vi "background writer.vi"(0 "dictionary":T1, 1 "command queue":refnum<k33>, 2 "response from processor":refnum<k33>, 3 "output type order":T3[](array[typedef]), 5 "logging path":path, 7 "backup directory":path, 9 "cache allocation":T2, 10 "LogRotate":refnum<class "LogRotate.lvclass">=refnum, 11 "scans per write":u16=20, 12 "dictionary group names":T1, 13 "enable channel (bool)":i32, 14 "has enable channel":bool) -> (15 "error out":errorcluster)   [LabVIEW 2015, in "TDMS datalogger runtime.lvclass"]
uses:
  TDMS datalogger runtime.lvclass
  <vilib>/NI/Tag Bus/tag/Data Type.ctl
  data cache.ctl
  <vilib>/NI/Tag Bus/dictionary/full data dictionary.ctl
  message to background process.ctl
  control enum.ctl
  <vilib>/NI/Tag Bus/table/data table.ctl
  response from background process.ctl
  response enum.ctl
  <vilib>/NI/LogRotate/LogRotate.lvclass
  writer state enum.ctl
  <vilib>/NI/Tag Bus/table/data table.lvlib
  <vilib>/NI/Tag Bus/tag/tag descriptor.lvclass
  <vilib>/NI/Tag Bus/dictionary/data dictionary.lvclass
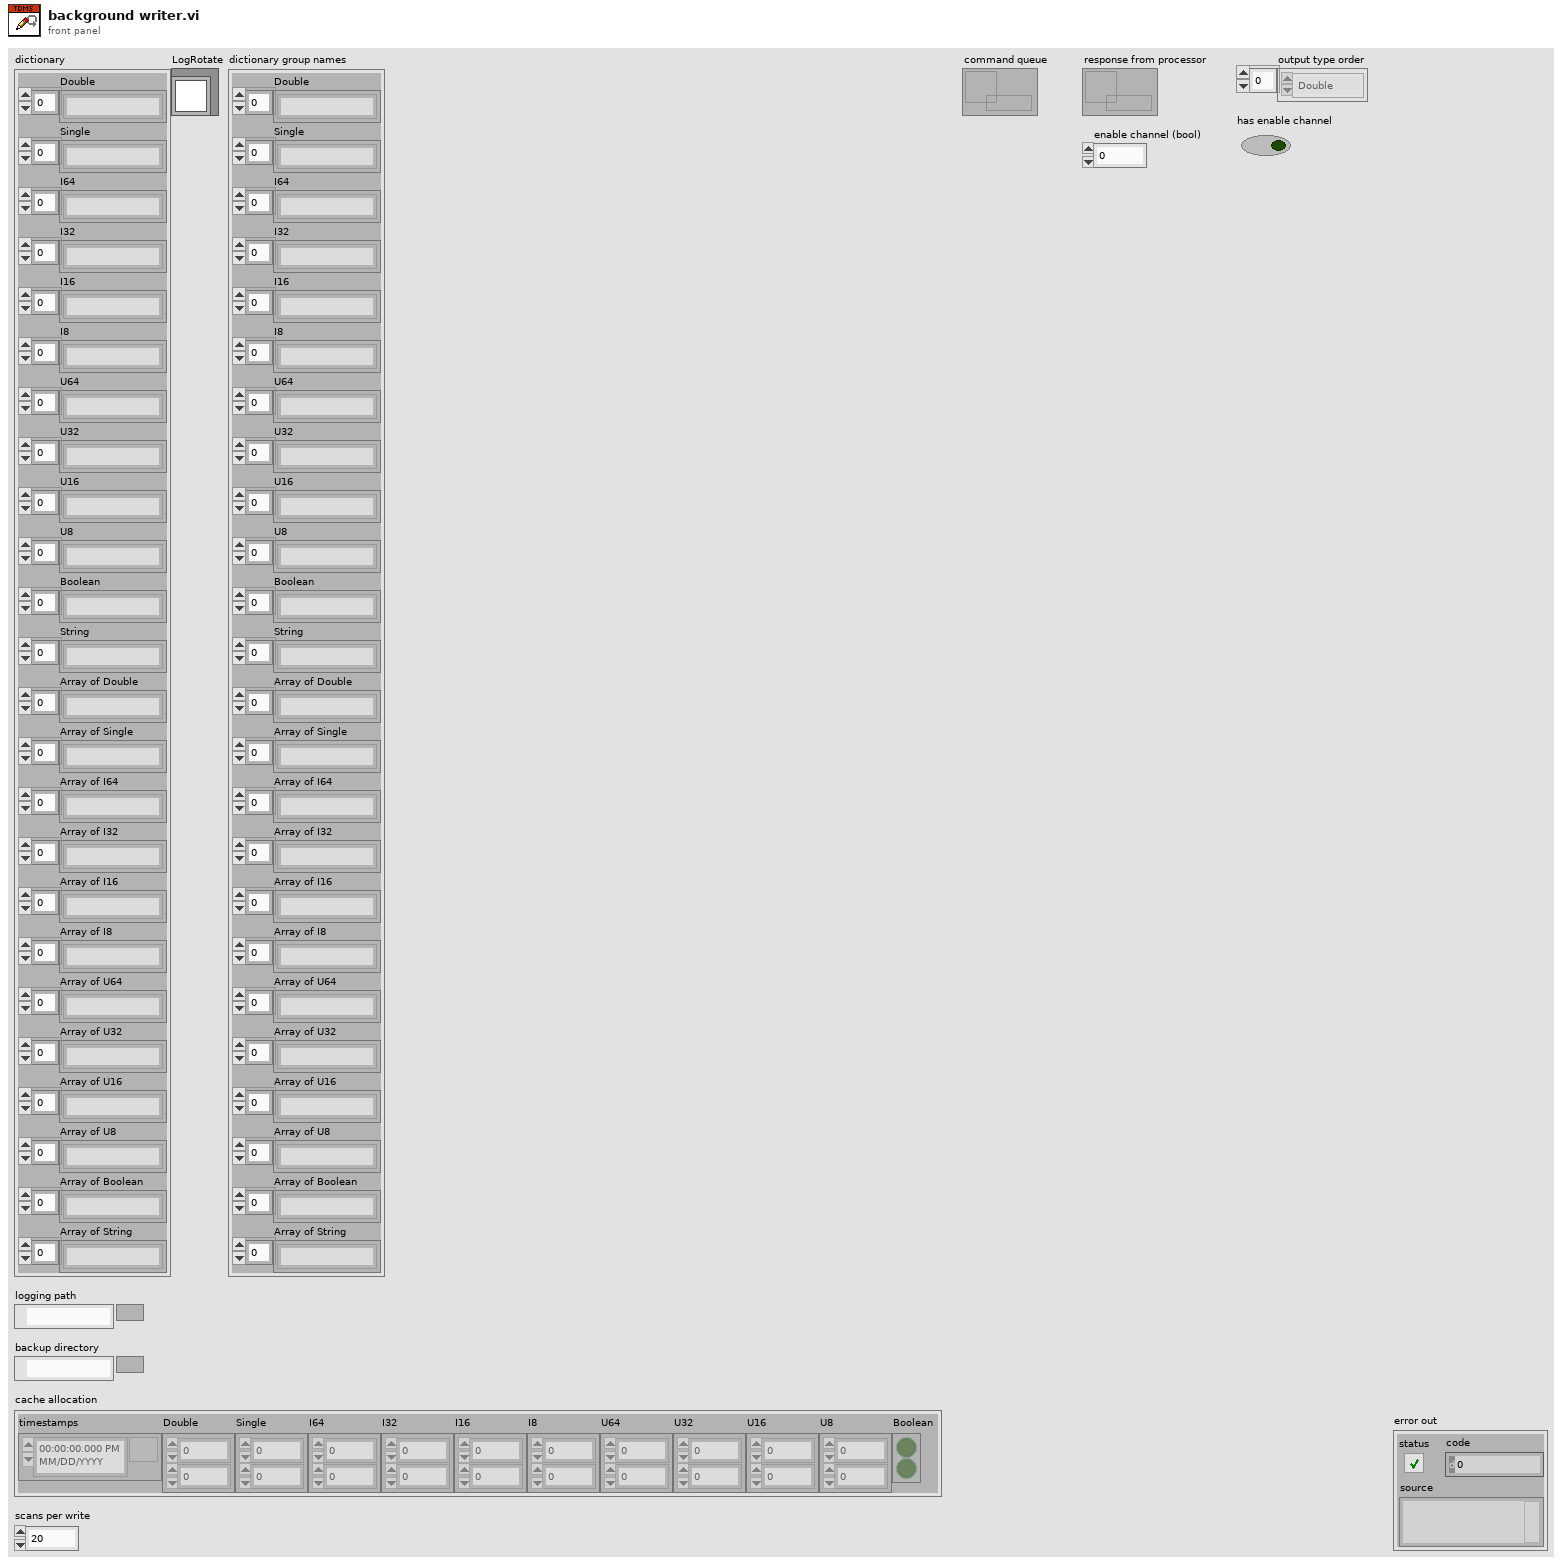
[diagram p1: front panel]
types:
  T1 = typedef "tag bus.lvlib/data dictionary.lvclass/full data dictionary.ctl" = cluster{"Double":string[], "Single":string[], "I64":string[], "I32":string[], "I16":string[], "I8":string[], "U64":string[], "U32":string[], "U16":string[], "U8":string[], "Boolean":string[], "String":string[], "Array of Double":string[], "Array of Single":string[], "Array of I64":string[], "Array of I32":string[], "Array of I16":string[], "Array of I8":string[], "Array of U64":string[], "Array of U32":string[], "Array of U16":string[], "Array of U8":string[], "Array of Boolean":string[], "Array of String":string[]}
  T2 = typedef "TDMS datalogger runtime.lvclass/data cache.ctl" = cluster{"timestamps":timestamp[], "Double":dbl[][], "Single":sgl[][], "I64":i64[][], "I32":i32[][], "I16":i16[][], "I8":i8[][], "U64":u64[][], "U32":u32[][], "U16":u16[][], "U8":u8[][], "Boolean":bool[][]}
  T3 = typedef "tag bus.lvlib/tag descriptor.lvclass/Data Type.ctl" = enum16{"Double", "Single", "I64", "I32", "I16", "I8", "U64", "U32", "U16", "U8", "Boolean", "String", "Array of Double", "Array of Single", "Array of I64", "Array of I32", "Array of I16", "Array of I8", "Array of U64", "Array of U32", "Array of U16", "Array of U8", "Array of Boolean", "Array of String"}
  T4 = typedef "TDMS datalogger runtime.lvclass/writer state enum.ctl" = enum16{"wait for message", "report error", "exit", "close file"}
  T5 = typedef "TDMS datalogger runtime.lvclass/response enum.ctl" = enum16{"exit", "return buffer", "error"}
  T6 = typedef "TDMS datalogger runtime.lvclass/response from background process.ctl" = cluster{"response enum":T5, "datapack":refnum<data-value>, "error code":i32}
  T7 = typedef "TDMS datalogger runtime.lvclass/message to background process.ctl" = cluster{"control enum":T8, "datapack":refnum<data-value>, "Time Stamp":timestamp}
  T8 = typedef "TDMS datalogger runtime.lvclass/control enum.ctl" = enum16{"exit", "output data"}
  T9 = typedef "tag bus.lvlib/data table.lvlib/data table.ctl" = cluster{"Double":dbl[], "Single":sgl[], "I64":i64[], "I32":i32[], "I16":i16[], "I8":i8[], "U64":u64[], "U32":u32[], "U16":u16[], "U8":u8[], "Boolean":bool[], "String":string[], "Array of Double":cluster{"DBL Array":dbl[]}[], "Array of Single":cluster{"SGL Array":sgl[]}[], "Array of I64":cluster{"I64 Array":i64[]}[], "Array of I32":cluster{"I32 Array":i32[]}[], "Array of I16":cluster{"I16 Array":i16[]}[], "Array of I8":cluster{"I8 Array":i8[]}[], "Array of U64":cluster{"U64 Array":u64[]}[], "Array of U32":cluster{"U32 Array":u32[]}[], "Array of U16":cluster{"U16 Array":u16[]}[], "Array of U8":cluster{"U8 Array":u8[]}[], "Array of Boolean":cluster{"Boolean Array":bool[]}[], "Array of String":cluster{"String Array":string[]}[]}
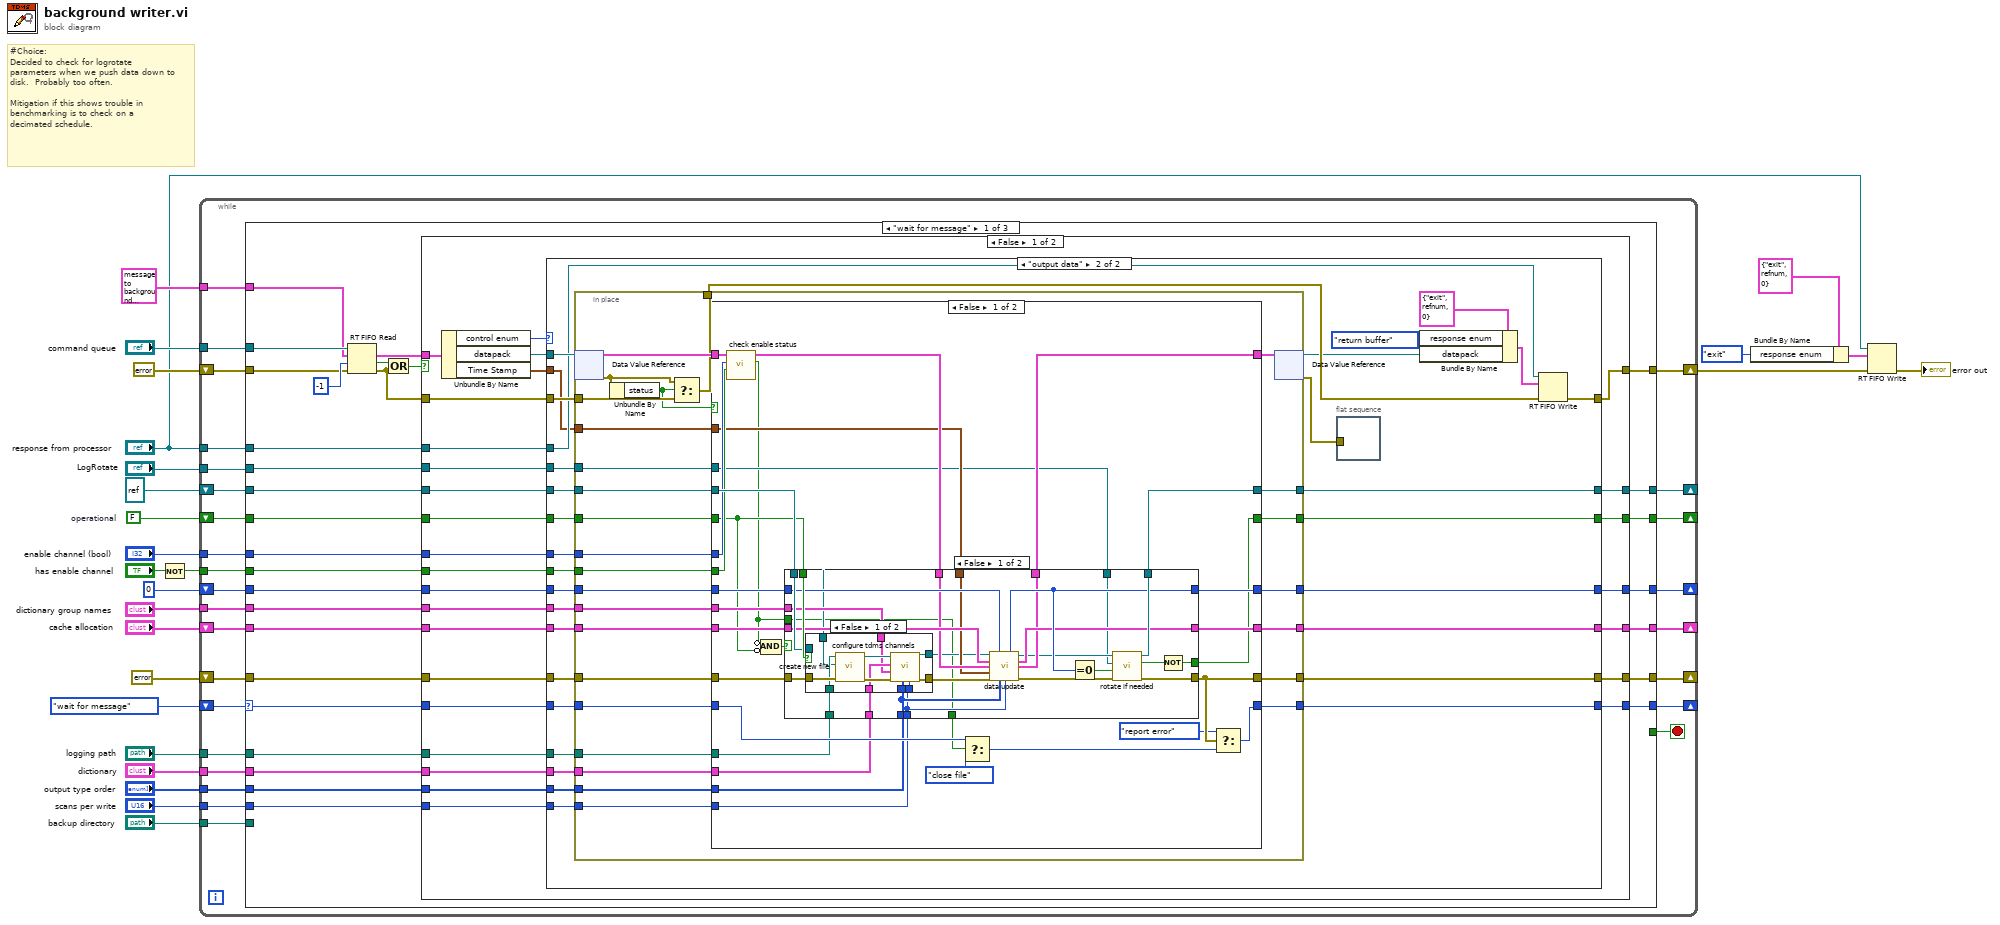
[diagram p0: block diagram]
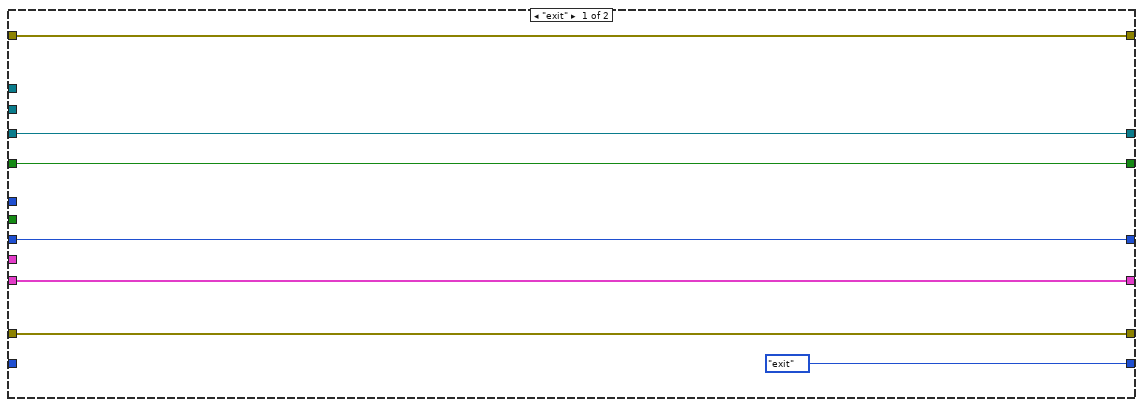
[diagram p2: hidden frame]
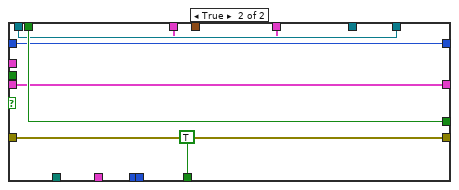
[diagram p4: hidden frame]
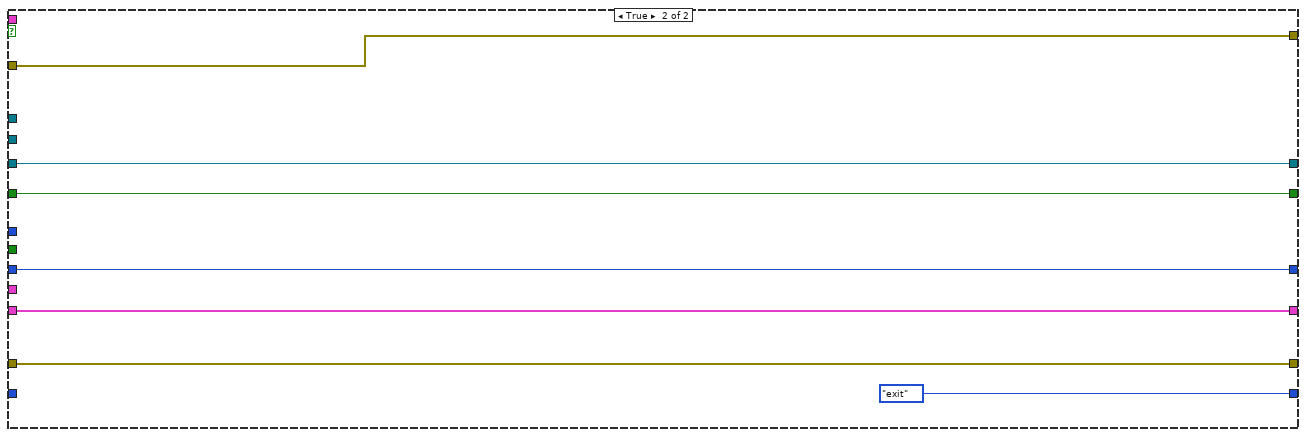
[diagram p6: hidden frame]
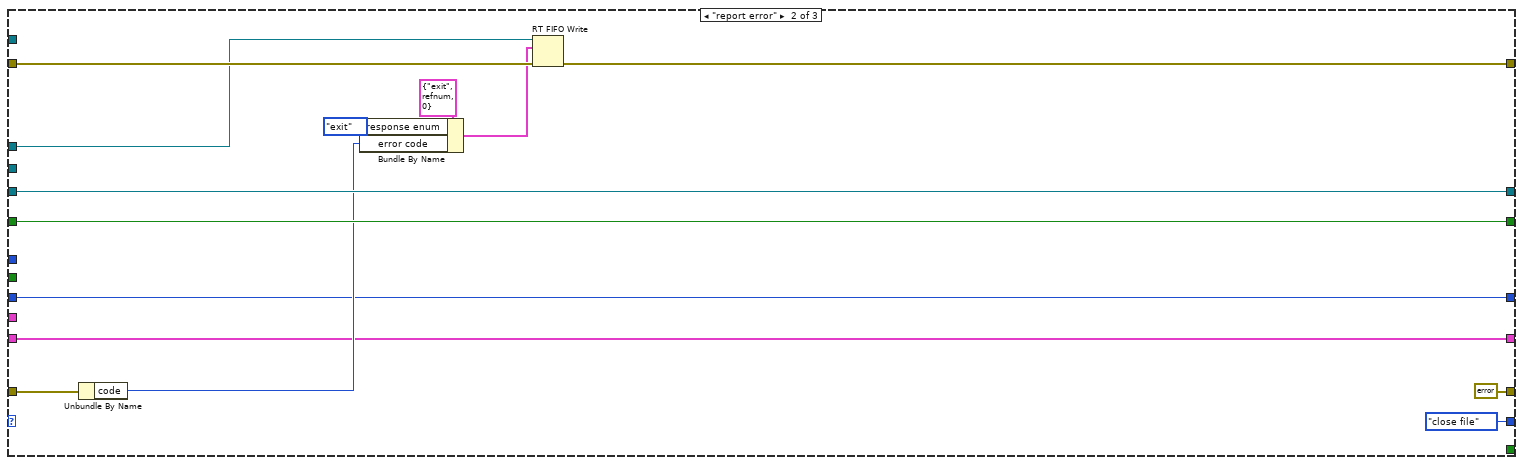
[diagram p7: hidden frame]
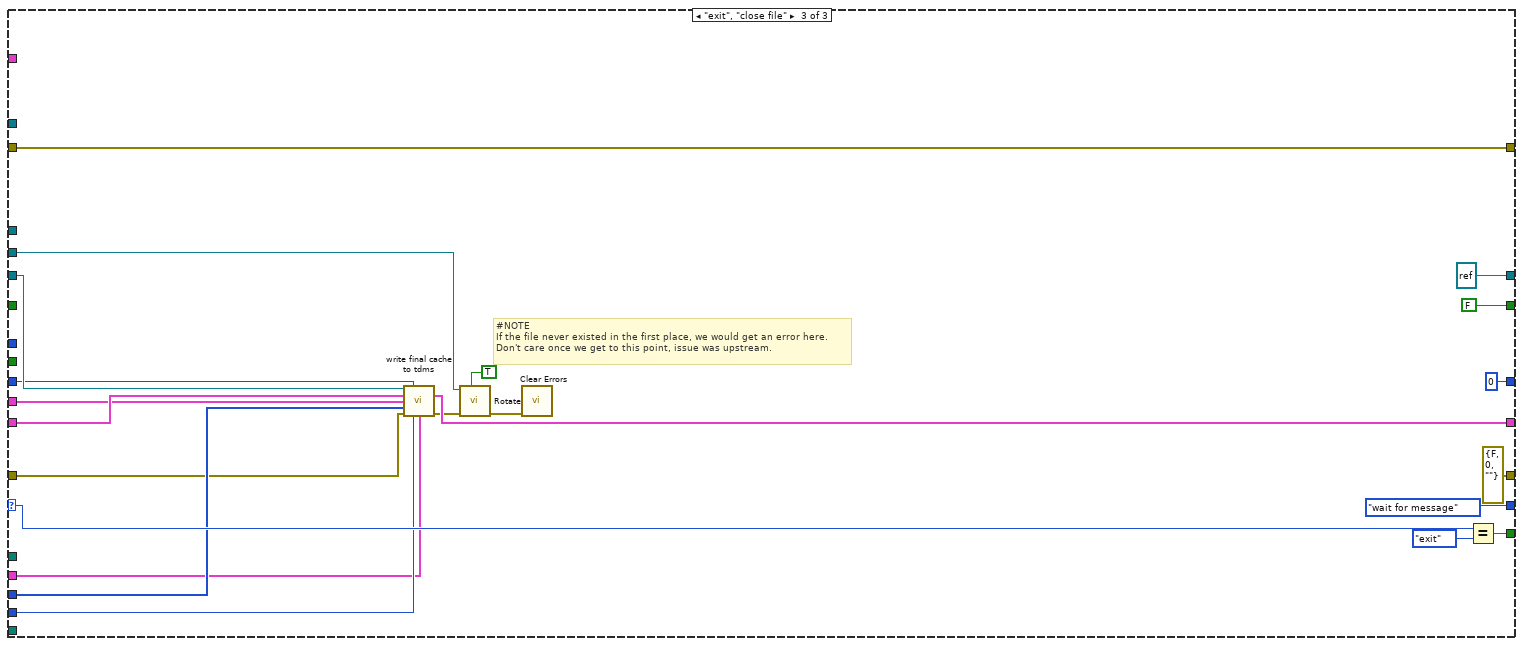
[diagram p8: hidden frame]
diagram:
  w14 = FALSE  # operational
  # "#Choice:\nDecided to check for logrotate parameters when we push data down to disk.  Probably too often.\n\nMitigation if this shows trouble in benchmarking is to check on a decimated schedule."
  n1 = Not(x="has enable channel") -> (.not. x?=w6:bool)
  n2 = while {
    tunnel: "command queue" -> [w52]
    tunnel: T7 {"control enum"=enum."exit", "datapack"=refnum, "Time Stamp"=timestamp(0 s since 1904-01-01)} ("element") -> [w51]
    shift-right: [w49] -> w22
    shift-left: errorcluster {"status"=FALSE, "code"=0, "source"=""} ("error in") -> [w50]
    tunnel: "response from processor" -> [w47]
    shift-right: [w45] -> _
    shift-left: writer_state_enum."wait for message" ("logger state") -> [w46]
    shift-right: [w43] -> _
    shift-left: refnum<k34> refnum ("tdms file out") -> [w44]
    shift-right: [w34] -> _
    shift-left: w14 -> [w42]
    shift-right: [w40] -> _
    shift-left: errorcluster {"status"=FALSE, "code"=0, "source"=""} ("error in") -> [w41]
    tunnel: "logging path" -> [w39]
    tunnel: "dictionary" -> [w38]
    tunnel: "output type order" -> [w37]
    tunnel: "scans per write" -> [w36]
    tunnel: "backup directory" -> [w35]
    shift-right: [w33] -> _
    shift-left: 0 ("sample counter") -> [w32]
    shift-right: [w27] -> _
    shift-left: "cache allocation" -> [w28]
    tunnel: "enable channel (bool)" -> [w30]
    tunnel: w6 -> [w31]
    tunnel: "dictionary group names" -> [w29]
    tunnel: "LogRotate" -> [w26]
    stop <- w48 stop-if-true
    n3 = case shown="\"wait for message\"" w46 {
      selector: w46 -> [w61 _ w298]
      tunnel: w52 -> [w82 _ _]
      tunnel: w51 -> [w80 _ _]
      tunnel: w50 -> [w79 w278 w300]
      tunnel: [w75 w276 w300] -> w49
      tunnel: [_ _ w299] -> w48
      tunnel: w47 -> [w73 w275 _]
      tunnel: [w72 writer_state_enum."close file" ("logger state") writer_state_enum."wait for message" ("logger state")] -> w45
      tunnel: w44 -> [w71 w277 w291]
      tunnel: [w70 w277 refnum<k34> refnum ("tdms file out")] -> w43
      tunnel: w42 -> [w68 w269 _]
      tunnel: w41 -> [w66 w268 w283]
      tunnel: [w67 errorcluster {"status"=FALSE, "code"=0, "source"=""} ("error out") errorcluster {"status"=FALSE, "code"=0, "source"=""} ("error out")] -> w40
      tunnel: w39 -> [w55 _ _]
      tunnel: w38 -> [w53 _ w285]
      tunnel: w37 -> [w58 _ w288]
      tunnel: w36 -> [w57 _ w286]
      tunnel: w35 -> [_ _ _]
      tunnel: [w69 w269 FALSE] -> w34
      tunnel: [w64 w265 0 ("sample counter")] -> w33
      tunnel: w32 -> [w65 w265 w287]
      tunnel: w31 -> [w59 _ _]
      tunnel: w30 -> [w60 _ _]
      tunnel: w29 -> [w54 _ w289]
      tunnel: w28 -> [w63 w266 w290]
      tunnel: [w62 w266 w284] -> w27
      tunnel: w26 -> [w56 _ w280]
      frame "wait for message" {
        n4 = RT FIFO Read(0:w82, 1:w80, 2:-1 ("timeout in ms (0)"), 3:w79) -> (9:w74:T7, 10:w78:bool, 11:w76:errorcluster)  [unwired: 2 out]
        n5 = Or(x=w78, y=w76) -> (x .or. y?=w77:bool)
        n6 = case shown="False" w77 {
          tunnel: w76 -> [w106 w264]
          tunnel: [w107 w264] -> w75
          tunnel: w74 -> [w109 _]
          tunnel: w73 -> [w103 _]
          tunnel: [w102 writer_state_enum."exit" ("logger state")] -> w72
          tunnel: w71 -> [w101 w262]
          tunnel: [w100 w262] -> w70
          tunnel: [w98 w261] -> w69
          tunnel: w68 -> [w99 w261]
          tunnel: [w97 w260] -> w67
          tunnel: w66 -> [w96 w260]
          tunnel: w65 -> [w94 w259]
          tunnel: [w95 w259] -> w64
          tunnel: w63 -> [w93 w258]
          tunnel: [w92 w258] -> w62
          tunnel: w61 -> [w91 _]
          tunnel: w60 -> [w90 _]
          tunnel: w59 -> [w89 _]
          tunnel: w58 -> [w88 _]
          tunnel: w57 -> [w87 _]
          tunnel: w56 -> [w86 _]
          tunnel: w55 -> [w85 _]
          tunnel: w54 -> [w84 _]
          tunnel: w53 -> [w83 _]
          frame False {
            n7 = Unbundle By Name(w109) -> ("control enum"=w108:T8, "datapack"=w104:refnum<data-value>, "Time Stamp"=w105:timestamp)
            n8 = case shown="\"output data\"" w108 {
              tunnel: [w116 w131] -> w107
              tunnel: w106 -> [w116 w146]
              tunnel: w105 -> [_ w123]
              tunnel: w104 -> [_ w147]
              tunnel: w103 -> [_ w128]
              tunnel: [writer_state_enum."exit" ("logger state") w135] -> w102
              tunnel: w101 -> [w114 w145]
              tunnel: [w114 w144] -> w100
              tunnel: w99 -> [w113 w142]
              tunnel: [w113 w143] -> w98
              tunnel: [w112 w136] -> w97
              tunnel: w96 -> [w112 w137]
              tunnel: [w110 w140] -> w95
              tunnel: w94 -> [w110 w141]
              tunnel: w93 -> [w111 w138]
              tunnel: [w111 w139] -> w92
              tunnel: w91 -> [_ w134]
              tunnel: w90 -> [_ w133]
              tunnel: w89 -> [_ w132]
              tunnel: w88 -> [_ w122]
              tunnel: w87 -> [_ w121]
              tunnel: w86 -> [_ w120]
              tunnel: w85 -> [_ w119]
              tunnel: w84 -> [_ w118]
              tunnel: w83 -> [_ w117]
              frame "exit" {
              }
              frame "output data" {
                n9 = in-place {
                  in-place-border: w146 -> [w174]
                  in-place-border: w145 -> [w169]
                  in-place-border: [w168] -> w144
                  in-place-border: [w167] -> w143
                  in-place-border: w142 -> [w166]
                  in-place-border: w141 -> [w165]
                  in-place-border: [w164] -> w140
                  in-place-border: [w163] -> w139
                  in-place-border: w138 -> [w162]
                  in-place-border: w137 -> [w161]
                  in-place-border: [w160] -> w136
                  in-place-border: [w159] -> w135
                  in-place-border: w134 -> [w158]
                  in-place-border: [w157] -> w130
                  in-place-border: w133 -> [w156]
                  in-place-border: w132 -> [w155]
                  in-place-border: w123 -> [w154]
                  in-place-border: w122 -> [w153]
                  in-place-border: w121 -> [w152]
                  in-place-border: w120 -> [w151]
                  in-place-border: w119 -> [w150]
                  in-place-border: w118 -> [w149]
                  in-place-border: w117 -> [w148]
                  n10 = in-place-dvr #1(w147) -> (w170:T9, w173:errorcluster)
                  n11 = Unbundle By Name(w173) -> ("status"=w172:bool)
                  n12 = Select(t=w173, s=w172, f=w174) -> (s? t:f=w157:errorcluster)
                  n13 = case shown="False" w172 {
                    tunnel: [w192 w257] -> w171
                    tunnel: w170 -> [w194 w257]
                    tunnel: w169 -> [w203 w256]
                    tunnel: [w204 w256] -> w168
                    tunnel: [w180 w255] -> w167
                    tunnel: w166 -> [w177 w255]
                    tunnel: w165 -> [w201 w254]
                    tunnel: [w202 w254] -> w164
                    tunnel: [w197 w253] -> w163
                    tunnel: w162 -> [w198 w253]
                    tunnel: w161 -> [w200 w252]
                    tunnel: [w199 w252] -> w160
                    tunnel: [w196 w251] -> w159
                    tunnel: w158 -> [w195 w251]
                    tunnel: w156 -> [w191 _]
                    tunnel: w155 -> [w190 _]
                    tunnel: w154 -> [w189 _]
                    tunnel: w153 -> [w188 _]
                    tunnel: w152 -> [w187 _]
                    tunnel: w151 -> [w179 _]
                    tunnel: w150 -> [w186 _]
                    tunnel: w149 -> [w185 _]
                    tunnel: w148 -> [w184 _]
                    frame False {
                      n14 = call "check enable status.vi"("always enabled?"=w190, "enable channel index"=w191, "data table in"=w194) -> ("enabled?"=w176:bool, "Data table out"=w193:T9)  [unwired: 7 in]
                      n15 = Compound Arithmetic op=AND(invert w176, invert w177) -> (w178:bool)
                      n16 = case shown="False" w178 {
                        tunnel: w177 -> [w230 w249]
                        tunnel: [w229 w247] -> w204
                        tunnel: w203 -> [w228 w247]
                        tunnel: [w227 w248] -> w202
                        tunnel: w201 -> [w226 w248]
                        tunnel: w200 -> [w225 w250]
                        tunnel: [w224 w250] -> w199
                        tunnel: w198 -> [w223 w246]
                        tunnel: [w222 w246] -> w197
                        tunnel: w193 -> [w221 w245]
                        tunnel: [w220 w245] -> w192
                        tunnel: w189 -> [w219 _]
                        tunnel: w188 -> [w218 _]
                        tunnel: w187 -> [w217 _]
                        tunnel: w186 -> [w216 _]
                        tunnel: w185 -> [w215 _]
                        tunnel: w184 -> [w214 _]
                        tunnel: [w207 w249] -> w180
                        tunnel: w179 -> [w206 _]
                        tunnel: w176 -> [w205 _]
                        tunnel: [w205 TRUE ("enabled?")] -> w175
                        frame False {
                          n17 = case shown="False" w230 {
                            tunnel: w228 -> [_ w242]
                            tunnel: w225 -> [w239 w243]
                            tunnel: [w238 w243] -> w210
                            tunnel: [w237 w242] -> w209
                            tunnel: w216 -> [w236 _]
                            tunnel: w215 -> [w231 _]
                            tunnel: w214 -> [w235 _]
                            tunnel: w218 -> [w234 _]
                            tunnel: w217 -> [w233 _]
                            tunnel: w206 -> [w232 _]
                            frame False {
                              n18 = call "create new file.vi"("error in"=w239, "LogRotate in"=w232, "logging path"=w236) -> ("error out"=w241:errorcluster, "tdms file out"=w240:refnum<k34>)  [unwired: 7 in]
                              n19 = call "configure tdms channels.vi"("samples per channel (1)"=w233, "type order"=w234, "error in"=w241, "dictionary group names"=w231, "dictionary"=w235, "tdms file in"=w240) -> ("error out"=w238:errorcluster, "tdms file out"=w237:refnum<k34>)  [unwired: 4 in]
                            }
                            frame True {
                            }
                          }
                          n20 = call "data update.vi"("tdms in"=w209, "sample counter in"=w226, "cache in"=w223, "data table in"=w221, "Time Stamp"=w219, "error in"=w210, "output type order"=w218, "scans per write"=w217) -> ("sample counter out"=w227:i32, "tdms out"=w212:refnum<k34>, "cache out"=w222:T2, "data table out"=w220:T9, "error out"=w213:errorcluster)  [unwired: 3 in]
                          n21 = Equal To 0?(x=w227) -> (x = 0?=w211:bool)
                          n22 = call "rotate if needed.vi"("error in"=w213, "Check?"=w211, "LogRotate"=w206, "tdms ref in"=w212) -> ("error out"=w224:errorcluster, "rotated?"=w208:bool, "tdms ref out"=w229:refnum<k34>)  [unwired: 5 in]
                          n23 = Not(x=w208) -> (.not. x?=w207:bool)
                        }
                        frame True {
                        }
                      }
                      n24 = Select(t=w195, s=w175, f=writer_state_enum."close file") -> (s? t:f=w181:T4)
                      n25 = Select(t=writer_state_enum."report error", s=w199, f=w181) -> (s? t:f=w196:T4)
                    }
                    frame True {
                    }
                  }
                  n26 = in-place-dvr #1(w171) -> (w125:refnum<data-value>, w129:errorcluster)
                }
                n27 = flat-sequence {
                  tunnel: w129 -> [_]
                  frame #0 {
                  }
                }
                n28 = Bundle By Name(cluster=T6 {"response enum"=enum."exit", "datapack"=refnum, "error code"=0} ("element"), "response enum"=response_enum."return buffer", "datapack"=w125) -> (w126:T6)
                n29 = RT FIFO Write(0:w128, 1:w126, 3:w130) -> (11:w131:errorcluster)  [unwired: 2 in, 3 out]
              }
            }
          }
          frame True {
          }
        }
      }
      frame "report error" {
        n30 = Unbundle By Name(w268) -> ("code"=w267:i32)
        n31 = Bundle By Name(cluster=T6 {"response enum"=enum."exit", "datapack"=refnum, "error code"=0} ("element"), "response enum"=response_enum."exit", "error code"=w267) -> (w273:T6)
        n32 = RT FIFO Write(0:w275, 1:w273, 3:w278) -> (11:w276:errorcluster)  [unwired: 2 in, 3 out]
      }
      frame "exit", "close file" {
        # "#NOTE\nIf the file never existed in the first place, we would get an error here.\nDon't care once we get to this point, issue was upstream."
        n33 = call "write final cache to tdms.vi"("tdms file in"=w291, "sample counter"=w287, "cache in"=w290, "dictionary group names"=w289, "output type order"=w288, "error in"=w283, "scans per write"=w286, "dictionary"=w285) -> ("cache out"=w284:T2, "error out"=w282:errorcluster)  [unwired: 6 in]
        n34 = call <vilib>:"Rotate.vi"("Force rotate"=TRUE, "error in (no error)"=w282, "LogRotate in"=w280) -> ("error out"=w281:errorcluster)  [unwired: 7 in, 1 out]
        n35 = call <vilib>:"Clear Errors.vi"("error in (no error)"=w281) -> ()  [unwired: 5 in, 2 out]
        n36 = Equal?(x=w298, y=writer_state_enum."exit") -> (x = y?=w299:bool)
      }
    }
  }
  n37 = Bundle By Name(cluster=T6 {"response enum"=enum."exit", "datapack"=refnum, "error code"=0} ("element"), "response enum"=response_enum."exit") -> (w19:T6)
  n38 = RT FIFO Write(0:"response from processor", 1:w19, 3:w22) -> (11:→"error out":errorcluster)  [unwired: 2 in, 3 out]
